vi "Add Tab.vi"(8 "error in":errorcluster, 11 "Tab Control Reference In":refnum<vi>) -> (0 "error out":errorcluster, 3 "Tab Control Reference Out":refnum<vi>)   [LabVIEW 2017, in "DTacq Plot Display Library.lvlib"]
doc: "Prepares the graphical user interface for display;\nGUI controls are set to their default values,\nThe front panel is centered on the screen,\nThe front panel is opened, if not already open"
uses:
  DTacq Plot Display Library.lvlib
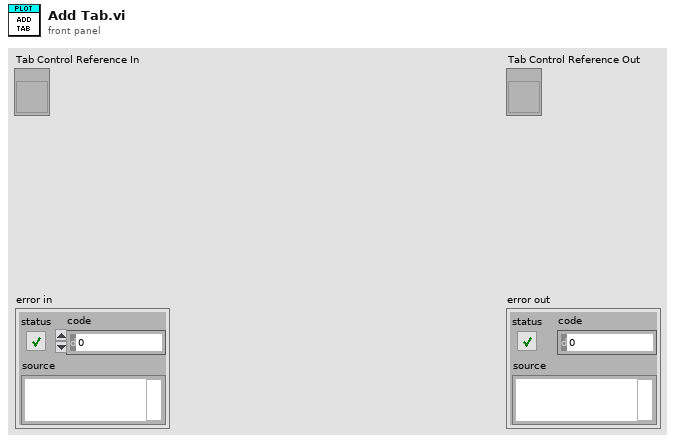
[diagram p1: front panel]
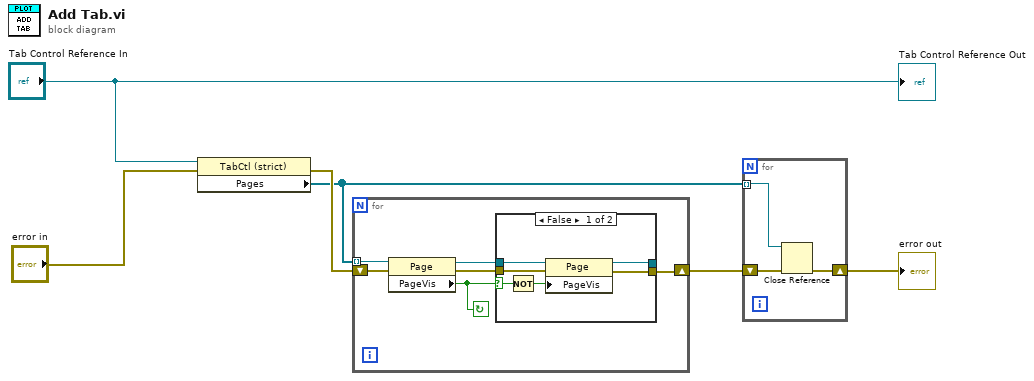
[diagram p0: block diagram]
diagram:
  n1 = property class="TabCtl (strict)"(reference="Tab Control Reference In", error in="error in") -> (error out=w4:errorcluster, "Pages"=w1:refnum<vi>[])  [unwired: 1 out]
  n2 = for {
    tunnel: w1 -> [w12] mode=indexing
    shift-right: [w7] -> w3
    shift-left: w4 -> [w11]
    stop <- w8 continue-if-true
    n3 = property class="Page"(reference=w12, error in=w11) -> (reference out=w10:refnum<vi>, error out=w9:errorcluster, "PageVis"=w8:bool)
    n4 = case shown="False" w8 {
      selector: w8 -> [w18 _]
      tunnel: w10 -> [w16 w20]
      tunnel: w9 -> [w15 w19]
      tunnel: [w14 w20] -> _
      tunnel: [w13 w19] -> w7
      frame False {
        n5 = Not(x=w18) -> (.not. x?=w17:bool)
        n6 = property class="Page"(reference=w16, error in=w15, "PageVis"=w17) -> (reference out=w14:refnum<vi>, error out=w13:errorcluster)
      }
      frame True {
      }
    }
  }
  n7 = for {
    shift-right: [w22] -> w2
    shift-left: w3 -> [w23]
    tunnel: w1 -> [w21] mode=indexing
    n8 = Close Reference(reference=w21, error in (no error)=w23) -> (error out=w22:errorcluster)
  }
  "error out" <- w2
  "Tab Control Reference Out" <- "Tab Control Reference In"
